vi "Keyin Field.vi"() -> (0 "Magnetic Field  value":dbl format="%.2f")   [LabVIEW 2021]
panel:
  in  "Input Magnetic Field":dbl format="%.2f"
  in  "?":bool
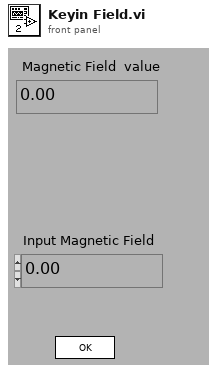
[diagram p1: front panel]
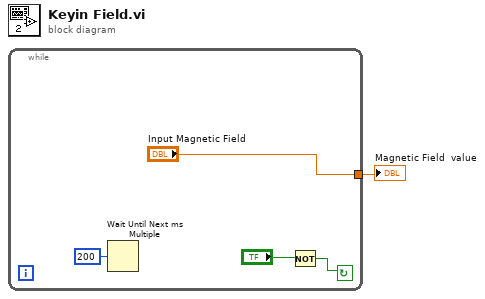
[diagram p0: block diagram]
diagram:
  n1 = while {
    tunnel: ["Input Magnetic Field"] -> w1
    stop <- w2 continue-if-true
    n2 = Wait Until Next ms Multiple(millisecond multiple=u32 200) -> ()  [unwired: 1 out]
    n3 = Not(x="?") -> (.not. x?=w2:bool)
  }
  "Magnetic Field  value" <- w1
